vi "Eulogy User.vi"(11 "Label Text":string) -> (3 "User":string)   [LabVIEW 2018, in "Bookmark Manager.lvlib"]
uses:
  Bookmark Manager.lvlib
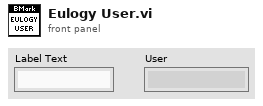
[diagram p1: front panel]
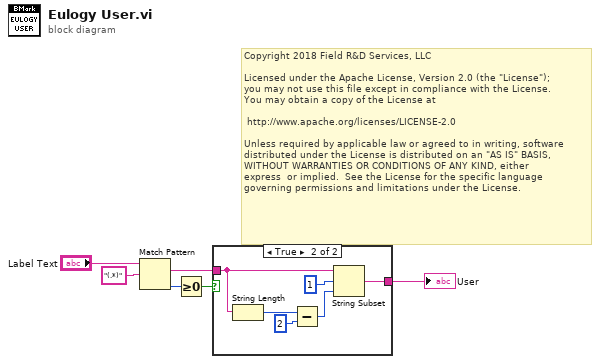
[diagram p0: block diagram]
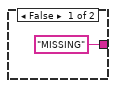
[diagram p2: hidden frame]
diagram:
  # "Copyright 2018 Field R&D Services, LLC\n\nLicensed under the Apache License, Version 2.0 (the \"License\");\nyou may not use this file except in compliance with the License.\nYou may obtain a copy of the License at\n\n\thttp://www.apache.org/licenses/LICENSE-2.0\n\nUnless required by applicable law or agreed to in writing, software\ndistributed under the License is distributed on an \"AS IS\" BASIS,\nWITHOUT WARRANTIES OR CONDITIONS OF ANY KIND, either \nexpress  or implied.  See the License for the specific language \ngoverning permissions and limitations under the License."
  n1 = Match Pattern(string="Label Text", regular expression="(.*)") -> (match substring=w5:string, offset past match=w2:i32)  [unwired: 1 in, 2 out]
  n2 = Greater Or Equal To 0?(x=w2) -> (x >= 0?=w1:bool)
  n3 = case shown="True" w1 {
    tunnel: ["MISSING" ("Label Text") w13] -> w6
    tunnel: w5 -> [_ w12]
    frame False {
    }
    frame True {
      n4 = String Length(string=w12) -> (length=w9:i32)
      n5 = Subtract(x=w9, y=2) -> (x-y=w11:i32)
      n6 = String Subset(string=w12, offset (0)=1, length (rest)=w11) -> (substring=w13:string)
    }
  }
  "User" <- w6
